vi "Ramp Once AB.vi"(4 "start ramp":bool, 6 "RT Loop Time (us)":i64, 7 "Voltage range":T3={"Vmax"=2700, "Vmin"=1800}, 8 "Total Ramp Time (us)":i64, 9 "down ramp multiplier":i32=3, 10 "Parameters In":T1={"Ramp State"=enum."intialize", "Ramp dV"=65535, "Ramp Voltage"=1350}) -> (2 "Parameters Out":T1={"Ramp State"=enum."intialize", "Ramp dV"=65535, "Ramp Voltage"=1350}, 3 "Measuring?":bool)   [LabVIEW 2018]
uses:
  Type Defs/voltage range.ctl
  Type Defs/ramp parameters.ctl
  Type Defs/ramp states.ctl
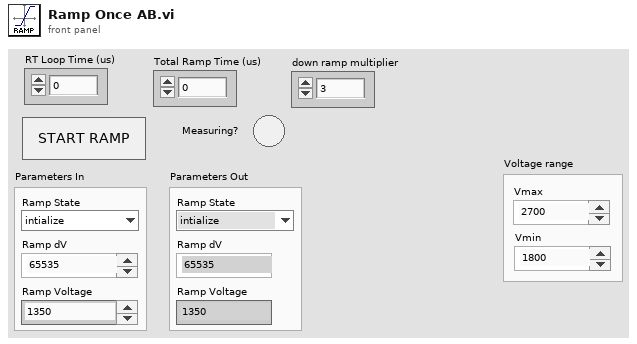
[diagram p1: front panel]
types:
  T1 = typedef "ramp parameters.ctl" = cluster{"Ramp State":T2, "Ramp dV":u16, "Ramp Voltage":u16}
  T2 = typedef "ramp states.ctl" = enum16{"intialize", "Ramp Down", "ramp up", "max"}
  T3 = typedef "voltage range.ctl" = cluster{"Vmax":u16, "Vmin":u16}
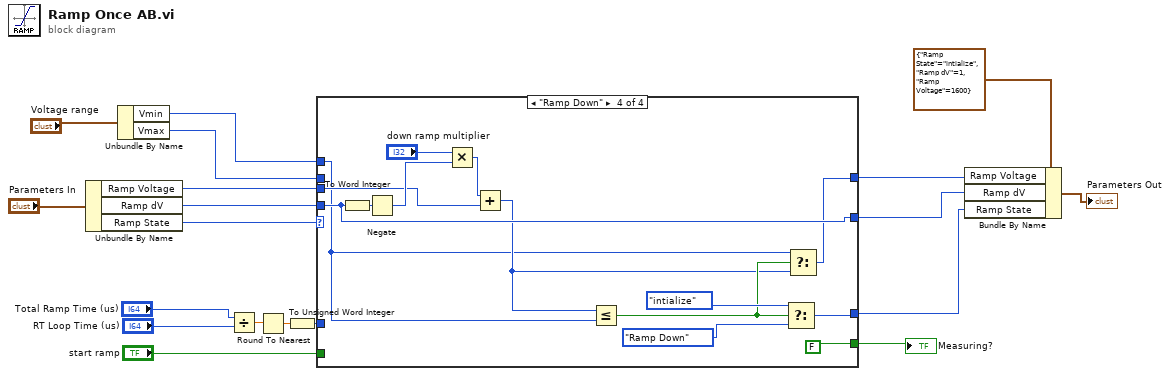
[diagram p0: block diagram]
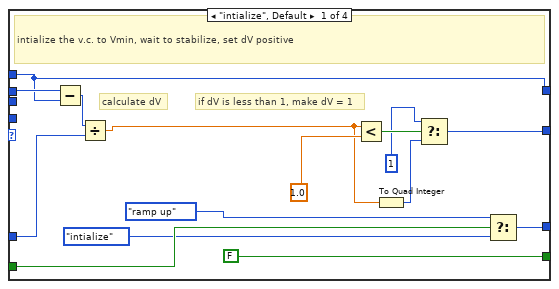
[diagram p2: hidden frame]
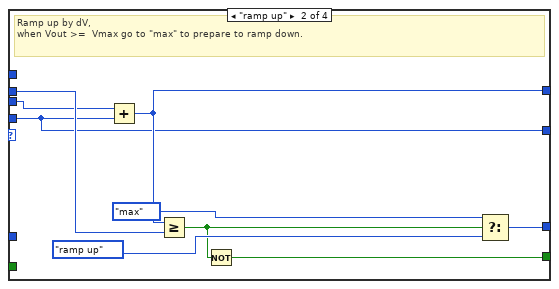
[diagram p3: hidden frame]
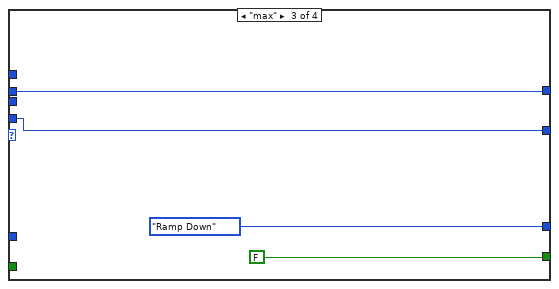
[diagram p4: hidden frame]
diagram:
  n1 = Unbundle By Name("Parameters In") -> ("Ramp Voltage"=w3:u16, "Ramp dV"=w4:u16, "Ramp State"=w5:T2)
  n2 = Unbundle By Name("Voltage range") -> ("Vmin"=w12:u16, "Vmax"=w11:u16)
  n3 = Divide(x="Total Ramp Time (us)", y="RT Loop Time (us)") -> (x/y=w19:dbl)
  n4 = Round To Nearest(number=w19) -> (nearest integer value=w18:dbl)
  n5 = To Unsigned Word Integer(number=w18) -> (unsigned 16bit integer=w17:u16)
  n6 = case shown="\"Ramp Down\"" w5 {
    tunnel: [w22 w35 w44 w52] -> w8
    tunnel: w11 -> [w33 w43 w47 _]
    tunnel: [w34 w42 ramp_states."Ramp Down" w58] -> w1
    tunnel: w12 -> [w29 _ _ w49]
    tunnel: w17 -> [w32 _ _ _]
    tunnel: "start ramp" -> [w30 _ _ _]
    tunnel: [w29 w41 w47 w48] -> w7
    tunnel: [FALSE w37 FALSE FALSE] -> w15
    tunnel: w4 -> [_ w35 w44 w52]
    tunnel: w3 -> [_ w36 _ w53]
    frame "intialize", Default {
      # "if dV is less than 1, make dV = 1"
      # "calculate dV"
      # "intialize the v.c. to Vmin, wait to stabilize, set dV positive"
      n7 = Subtract(x=w33, y=w29) -> (x-y=w31:u16)
      n8 = Divide(x=w31, y=w32) -> (x/y=w20:dbl)
      n9 = Less?(x=w20, y=1.0) -> (x < y?=w25:bool)
      n10 = To Quad Integer(1:w20) -> (0:w21:i64)
      n11 = Select(t=1, s=w25, f=w21) -> (s? t:f=w22:i64)
      n12 = Select(t=ramp_states."ramp up", s=w30, f=ramp_states."intialize") -> (s? t:f=w34:T2)
    }
    frame "ramp up" {
      # "Ramp up by dV,\nwhen Vout >=  Vmax go to \"max\" to prepare to ramp down."
      n13 = Add(x=w36, y=w35) -> (x+y=w41:u16)
      n14 = Greater Or Equal?(x=w41, y=w43) -> (x >= y?=w38:bool)
      n15 = Not(x=w38) -> (.not. x?=w37:bool)
      n16 = Select(t=ramp_states."max", s=w38, f=ramp_states."ramp up") -> (s? t:f=w42:T2)
    }
    frame "max" {
    }
    frame "Ramp Down" {
      n17 = To Word Integer(number=w52) -> (16bit integer=w59:i16)
      n18 = Negate(x=w59) -> (-x=w56:i16)
      n19 = Multiply(x="down ramp multiplier", y=w56) -> (x*y=w54:i32)
      n20 = Add(x=w54, y=w53) -> (x+y=w50:i32)
      n21 = Less Or Equal?(x=w50, y=w49) -> (x <= y?=w51:bool)
      n22 = Select(t=ramp_states."intialize", s=w51, f=ramp_states."Ramp Down") -> (s? t:f=w58:T2)
      n23 = Select(t=w49, s=w51, f=w50) -> (s? t:f=w48:i32)
    }
  }
  "Measuring?" <- w15
  n24 = Bundle By Name(cluster=T1 {"Ramp State"=enum."intialize", "Ramp dV"=1, "Ramp Voltage"=1600} ("Parameters 2"), "Ramp Voltage"=w7, "Ramp dV"=w8, "Ramp State"=w1) -> (→"Parameters Out":T1)
